vi "Merge LSS Strings.vi"(10 "Merge String":string, 11 "LSS Before":string) -> (3 "LSS After":string)   [LabVIEW 2019, in "LSS.lvlib"]
doc: "Merge two LSS strings such that there is no overlap, and the highest priority properties are still applied properly.\n\n<b>Inputs:</b>\n<b>LSS Before</b> - Input the LSS string currently in memory.\n<b>Merge String</b> - The new LSS to be merged with the LSS Before string.\n<b> Error in</b> - Standard Error In terminal.\n\n<b>Outputs:</b>\n<b>LSS After</b> - Merged LSS sring.\n<b>Error Out</b> - Standard Error out terminal."
uses:
  LSS.lvlib
panel:
  out "Error out":errorcluster
  in  "Error in":errorcluster
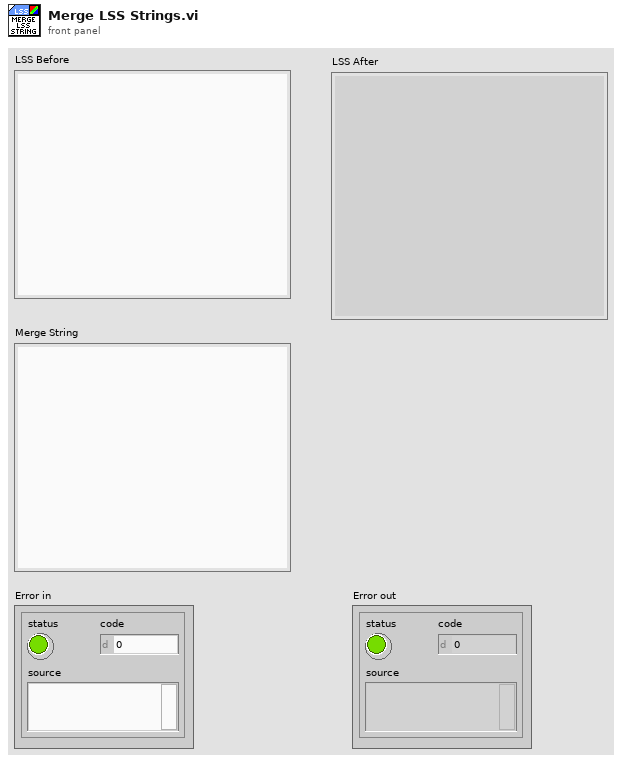
[diagram p1: front panel]
types:
  T1 = typedef "LSS.lvlib/Style.ctl" = cluster{"Specifier":string, "Properties":cluster{"Property":string, "Value":string}[]}
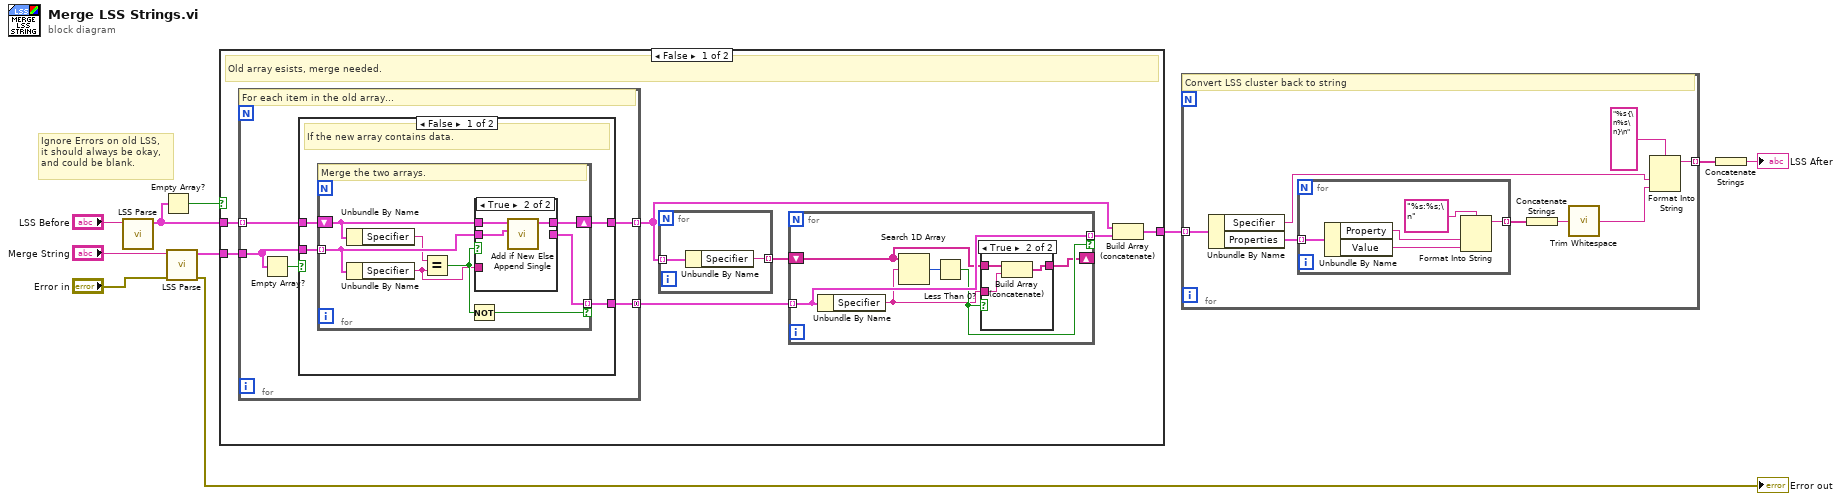
[diagram p0: block diagram]
diagram:
  # "Ignore Errors on old LSS,\nit should always be okay,\nand could be blank."
  n1 = call "LSS Parse.vi"("Style Sheet"="LSS Before") -> ("LSS Styles"=w4:T1[])  [unwired: 9 in, 1 out]
  n2 = Empty Array?(array=w4) -> (empty?=w3:bool)
  n3 = call "LSS Parse.vi"("Error in"="Error in", "Style Sheet"="Merge String") -> ("Error out"=→"Error out":errorcluster, "LSS Styles"=w8:T1[])  [unwired: 8 in]
  n4 = case shown="False" w3 {
    tunnel: w8 -> [w17 w53]
    tunnel: w4 -> [w16 _]
    tunnel: [w15 w53] -> w7
    frame False {
      # "Old array esists, merge needed."
      n5 = for {
        tunnel: w16 -> [w34] mode=indexing
        tunnel: w17 -> [w31]
        tunnel: [w33] -> w12 mode=indexing
        tunnel: [w32] -> w14 mode=concatenating
        # "For each item in the old array..."
        n6 = Empty Array?(array=w31) -> (empty?=w30:bool)
        n7 = case shown="False" w30 {
          tunnel: w34 -> [w38 w52]
          tunnel: w31 -> [w37 _]
          tunnel: [w36 w52] -> w33
          tunnel: [w35 _] -> w32
          frame False {
            # "If the new array contains data."
            n8 = for {
              shift-right: [w46] -> w36
              shift-left: w38 -> [w45]
              tunnel: w37 -> [w44] mode=indexing
              tunnel: [w42] -> w35 mode=indexing if=w40
              # "Merge the two arrays."
              n9 = Unbundle By Name(w45) -> ("Specifier"=w43:string)
              n10 = Unbundle By Name(w44) -> ("Specifier"=w39:string)
              n11 = Equal?(x=w43, y=w39) -> (x = y?=w41:bool)
              n12 = Not(x=w41) -> (.not. x?=w40:bool)
              n13 = case shown="True" w41 {
                tunnel: w45 -> [w48 w51]
                tunnel: w44 -> [w47 w50]
                tunnel: [w48 w49] -> w46
                tunnel: [w47 _] -> w42
                tunnel: w39 -> [_ _]
                frame False {
                }
                frame True {
                  n14 = call "Add if New Else Append Single.vi"("New Element"=w50, "Style In"=w51) -> ("Style Out"=w49:T1)  [unwired: 9 in]
                }
              }
            }
          }
          frame True {
            # "No items to add."
          }
        }
      }
      n15 = for {
        tunnel: w12 -> [w19] mode=indexing
        tunnel: [w18] -> w11 mode=indexing
        n16 = Unbundle By Name(w19) -> ("Specifier"=w18:string)
      }
      n17 = for {
        tunnel: w14 -> [w24] mode=indexing
        shift-right: [w21] -> _
        shift-left: w11 -> [w22]
        tunnel: [w24] -> w13 mode=indexing if=w23
        n18 = Unbundle By Name(w24) -> ("Specifier"=w20:string)
        n19 = Search 1D Array(1D array=w22, element=w20) -> (index of element=w25:i32)  [unwired: 1 in]
        n20 = Less Than 0?(x=w25) -> (x < 0?=w23:bool)
        n21 = case shown="True" w23 {
          tunnel: w22 -> [w26 w29]
          tunnel: [w26 w28] -> w21
          tunnel: w20 -> [_ w27]
          frame False {
          }
          frame True {
            n22 = Build Array (concatenate)(w29, w27) -> (w28:string[])
          }
        }
      }
      n23 = Build Array (concatenate)(w12, w13) -> (w15:T1[])
    }
    frame True {
      # "Array not found, all items are new."
    }
  }
  n24 = for {
    tunnel: w7 -> [w61] mode=indexing
    tunnel: [w55] -> w6 mode=indexing
    # "Convert LSS cluster back to string"
    n25 = Unbundle By Name(w61) -> ("Specifier"=w58:string, "Properties"=w60:cluster{"Property":string, "Value":string}[])
    n26 = for {
      tunnel: w60 -> [w66] mode=indexing
      tunnel: [w62] -> w57 mode=indexing
      n27 = Unbundle By Name(w66) -> ("Property"=w64:string, "Value"=w63:string)
      n28 = Format Into String(format string="%s:%s;\n", w64, w63) -> (resulting string=w62:string)  [unwired: 2 in, 1 out]
    }
    n29 = Concatenate Strings(w57) -> (w56:string)
    n30 = call <vilib>:"Trim Whitespace.vi"("string"=w56) -> ("trimmed string"=w54:string)  [unwired: 1 in]
    n31 = Format Into String(format string="%s{\n%s\n}\n", w58, w54) -> (resulting string=w55:string)  [unwired: 2 in, 1 out]
  }
  n32 = Concatenate Strings(w6) -> (→"LSS After":string)
